vi "04-nested_data_structures.vi"() -> ()   [LabVIEW 2018, in "LV2Julia_examples.lvlib"]
uses:
  LV2Julia_examples.lvlib
  LV2Julia_core/VIs/Server or client state.ctl
  LV2Julia_core/VIs/detailed error info.ctl
  LV2Julia_core/VIs/StackFrame.ctl
  LV2Julia_core/VIs/Commands.ctl
  c1a008e0-c205-4ae9-8ab0-5de19ea2baa8.vi
  c1a008e0-c205-4ae9-8ab0-5de19ea2baa8.vi/78d8e0ed-b3ed-426c-95b9-83093f6f1b2c.vi
  c1a008e0-c205-4ae9-8ab0-5de19ea2baa8.vi/78d8e0ed-b3ed-426c-95b9-83093f6f1b2c.vi/e3021c9a-7728-4898-8385-ad9514802a4f.vi
  c1a008e0-c205-4ae9-8ab0-5de19ea2baa8.vi/78d8e0ed-b3ed-426c-95b9-83093f6f1b2c.vi/a8876e75-3da6-480c-819d-014450441066.vi
  c1a008e0-c205-4ae9-8ab0-5de19ea2baa8.vi/78d8e0ed-b3ed-426c-95b9-83093f6f1b2c.vi/b71caa43-6187-49cc-9329-579afc04e290.vi
  LV2Julia_core/VIs/jl-scripts path.vi
  LV2Julia_core/VIs/check ID validity.vi
  LV2Julia_core/VIs/bindata_descr to JSON.vi
  LV2Julia_core/VIs/check cluster field names.vi
  LV2Julia_core/VIs/concat JSON.vi
  LV2Julia_core/VIs/build request.vi
  LV2Julia_core/VIs/Parse server response.vi
  LV2Julia_core/VIs/log jl exceptions.vi
  LV2Julia_core/LV2Julia_core.lvlib
panel:
  out "returned value":T1
  in  "Argument":T2={"text_data"="hm?", "num_data"={"factor"=2, "num_arr"=[3.14, 2.72, 1.62]}} {"num_data"."num_arr" format="%#.2f"}
  in  "next":bool
  out "detailed error info":T3
  out "current error":errorcluster
  out "final error":errorcluster
  out "short err code":u8
  in  "stop":bool
  out "ZMQ timeout":bool
  out "Julia script file path":path
  out "temporary script path":path
  out "Jl Server state":T5
  # "Here the same (nested) data structure for the argument and returned value: for simplicity only."
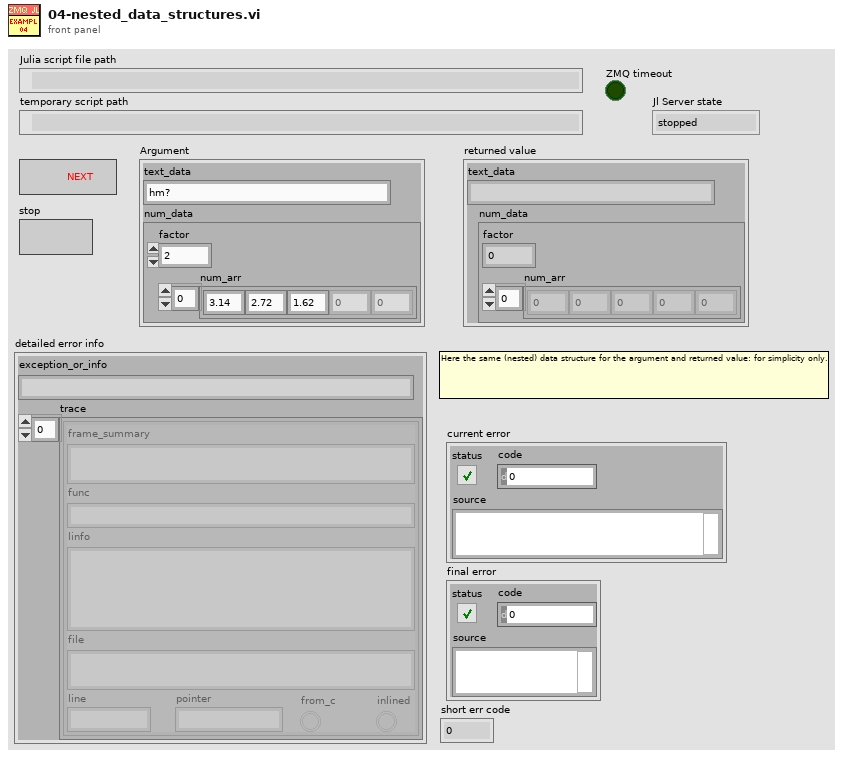
[diagram p1: front panel]
types:
  T1 = cluster{"text_data":string, "num_data":cluster{"factor":i32, "num_arr":dbl[]}}
  T2 = cluster{"text_data":string, "num_data":cluster{"factor":u32, "num_arr":dbl[]}}
  T3 = typedef "LV2Julia_core.lvlib/detailed error info.ctl" = cluster{"exception_or_info":string, "trace":T4[]}
  T4 = typedef "LV2Julia_core.lvlib/StackFrame.ctl" = cluster{"frame_summary":string, "func":string, "linfo":string, "file":string, "line":i32, "pointer":u64, "from_c":bool, "inlined":bool}
  T5 = typedef "LV2Julia_core.lvlib/Server or client state.ctl" = enum16{"stopped", "running", "unknown"}
  T6 = typedef "LV2Julia_core.lvlib/Commands.ctl" = enum16{"Start Jl-server & Init LV-client", "Send request & Get response ", "Stop Jl-server & Cleanup LV-client", "Cleanup LV-client", "Start Jl-server", "Stop Jl-server", "Init LV-Client", "Cleanup LV-Client", "(not allowed)", "Set LV Client state", "Set Jl Server state", "set ZMQ timeout", "read ZMQ timeout", "read-out state"}
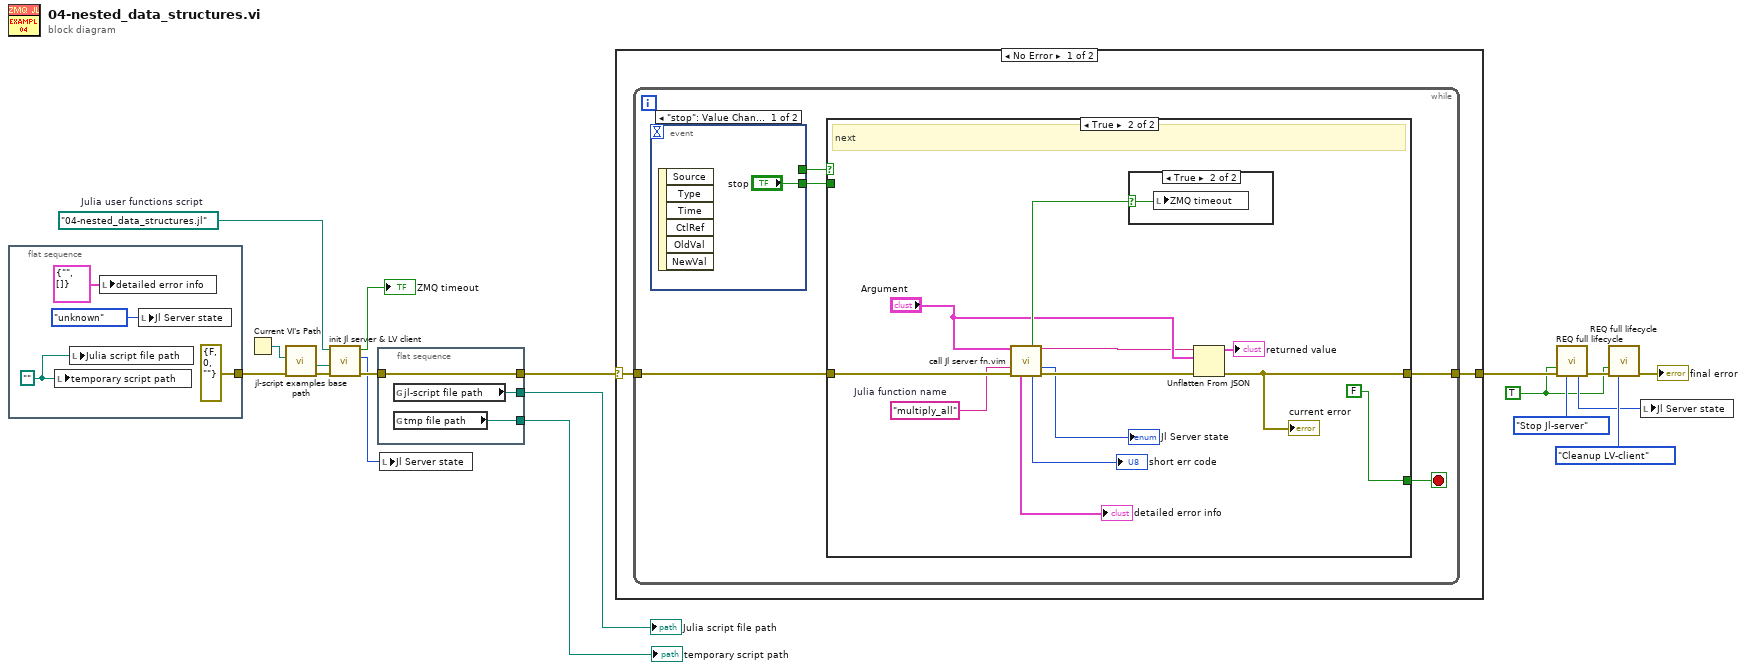
[diagram p0: block diagram]
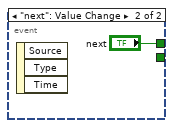
[diagram p2: hidden frame]
diagram:
  w5 = path "04-nested_data_structures.jl"  # Julia user functions script
  w9 = TRUE ("Force command")
  n1 = flat-sequence {
    tunnel: [errorcluster {"status"=FALSE, "code"=0, "source"=""} ("error in (no error)")] -> w1
    frame #0 {
      w19 = path ""
      n2 = local write "temporary script path"(w19) -> ()
      n3 = local write "Julia script file path"(w19) -> ()
      n4 = local write "detailed error info"(T3 {"exception_or_info"="", "trace"=[]} ("detailed error info")) -> ()
      n5 = local write "Jl Server state"(Server_or_client_state."unknown" ("Jl Server state out")) -> ()
    }
  }
  n6 = Current VI's Path() -> (path=w4:path)
  n7 = call "jl-script examples base path.vi"("error in (no error)"=w1, "calling example VI path"=w4) -> ("error out"=w3:errorcluster, "jl-script-examples base path"=w2:path)  [unwired: 8 in]
  n8 = call "init Jl server & LV client.vi"("error in (no error)"=w3, "Base path (not a path)"=w2, "Julia user functions script"=w5) -> ("error out"=w8:errorcluster, "Jl Server state out"=w6:T5, "timeout?"=→"ZMQ timeout":bool)  [unwired: 6 in]
  n9 = flat-sequence {
    tunnel: [w25] -> w13
    tunnel: w8 -> [w25]
    tunnel: [w24] -> w11
    tunnel: [w23] -> w12
    frame #0 {
      n10 = global read "jl-scripts path.vi" "jl-script file path"() -> (w24:path)
      n11 = global read "jl-scripts path.vi" "tmp file path"() -> (w23:path)
    }
  }
  n12 = local write "Jl Server state"(w6) -> ()
  n13 = case shown="No Error" w13 {
    selector: w13 -> [w26 w50]
    tunnel: [w27 w50] -> w18
    frame No Error {
      n14 = while {
        tunnel: w26 -> [w31]
        tunnel: [w32] -> w27
        stop <- w29 stop-if-true
        n15 = event shown="[0] \"stop\": Value Change" {
          selector: _ -> [_ _]
          dyn-events: _ -> [_ _]
          timeout: _ -> [_ _]
          tunnel: [_ "next"] -> w30
          tunnel: ["stop" _] -> w28
          event "stop": Value Change {
            n16 = event-data() -> ()  [unwired: 1 in, 6 out]
          }
          event "next": Value Change {
            n17 = event-data() -> ()  [unwired: 1 in, 3 out]
          }
        }
        n18 = case shown="True" w30 {
          tunnel: [w36 w47] -> w32
          tunnel: w31 -> [w36 w45]
          tunnel: [w35 FALSE ("stop this VI only")] -> w29
          tunnel: w28 -> [w35 _]
          frame False {
            # "stop"
          }
          frame True {
            w38 = "multiply_all"  # Julia function name
            # "next"
            n19 = call "call Jl server fn.vim"("Arguments 1"="Argument", "fun2call"=w38, "error in (no error)"=w45) -> ("timeout?"=w40:bool, "JSON received"=w37:string, "Jl Server state out"=→"Jl Server state":T5, "detailed error info"=→"detailed error info":T3, "return code"=→"short err code":u8, "error out"=w44:errorcluster)  [unwired: 6 in, 1 out]
            n20 = case shown="True" w40 {
              selector: w40 -> [_ w49]
              frame False {
              }
              frame True {
                n21 = local write "ZMQ timeout"(w49) -> ()
              }
            }
            n22 = Unflatten From JSON(JSON string=w37, type and defaults="Argument", error in (no error)=w44) -> (value=→"returned value":T2, error out=w47:errorcluster)  [unwired: 4 in]
            "current error" <- w47
          }
        }
      }
    }
    frame Error {
    }
  }
  n23 = call "REQ full lifecycle.vi"("Force command"=w9, "error in"=w18, "command"=Commands."Stop Jl-server") -> ("Jl Server state out"=w10:T5, "error out"=w16:errorcluster)  [unwired: 6 in, 5 out]
  n24 = call "REQ full lifecycle.vi"("Force command"=w9, "error in"=w16, "command"=Commands."Cleanup LV-client") -> ("error out"=→"final error":errorcluster)  [unwired: 6 in, 6 out]
  n25 = local write "Jl Server state"(w10) -> ()
  "temporary script path" <- w12
  "Julia script file path" <- w11
